vi "UT_FFTW.vi"(7 "UT FFTW States":T1=enum."Transform", 11 "Array":sgl[][](array[numeric])) -> (0 "Error":bool, 3 "Results":sgl[][](array[numeric]))   [LabVIEW 2014]
uses:
  UT FFTW States.ctl
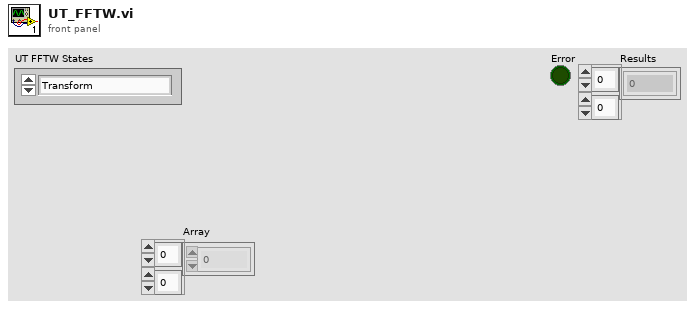
[diagram p1: front panel]
types:
  T1 = typedef "UT FFTW States.ctl" = enum16{"Init", "Transform", "Cleanup"}
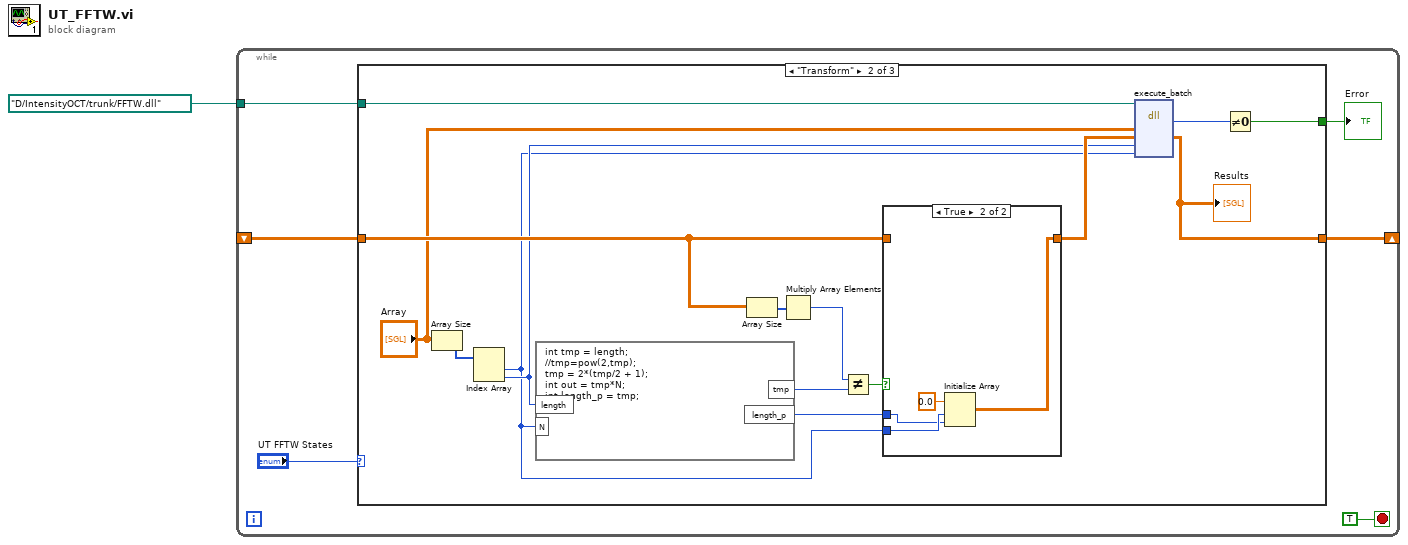
[diagram p0: block diagram]
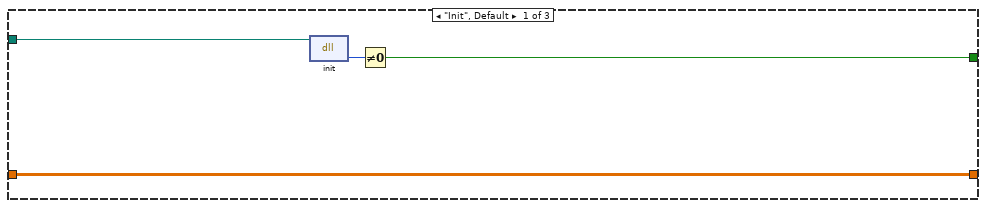
[diagram p2: hidden frame]
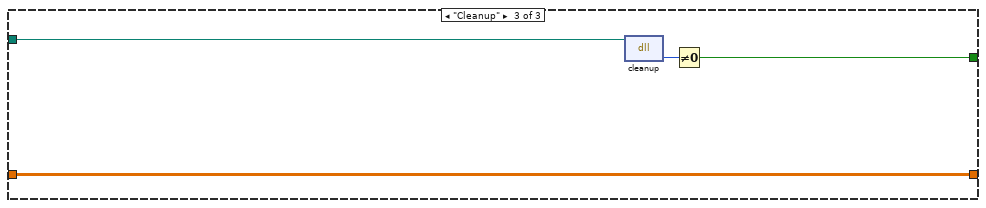
[diagram p4: hidden frame]
diagram:
  n1 = while {
    tunnel: path "D:/IntensityOCT/trunk/FFTW.dll" ("path in") -> [w5]
    shift-right: [w2] -> _
    shift-left: _ -> [w3]
    stop <- TRUE stop-if-true
    n2 = case shown="\"Transform\"" "UT FFTW States" {
      tunnel: w5 -> [w11 w19 w34]
      tunnel: [w9 w15 w32] -> w4
      tunnel: w3 -> [w8 w21 w35]
      tunnel: [w8 w14 w35] -> w2
      frame "Init", Default {
        n3 = dll-call lib="D:/IntensityOCT/trunk/FFT_CPP/x64/Release DLL/FFTW.dll" fn="init"(path in=w11) -> ("return type"=w10:i32)  [unwired: 2 in, 2 out]
        n4 = Not Equal To 0?(x=w10) -> (x != 0?=w9:bool)
      }
      frame "Transform" {
        n5 = Array Size(array="Array") -> (size(s)=w26:i32[])
        n6 = Index Array(array=w26) -> (element #1=w12:i32, element #2=w13:i32)  [unwired: 2 in]
        n7 = formula code="int tmp = length;\n//tmp=pow(2,tmp);\ntmp = 2*(tmp/2 + 1);\nint out = tmp*N;\nint length_p = tmp;"("length"=w13, "N"=w12) -> ("tmp"=w24:i32, "length_p"=w20:i32)
        n8 = Array Size(array=w21) -> (size(s)=w25:i32[])
        n9 = Multiply Array Elements(1:w25) -> (0:w23:i32)
        n10 = Not Equal?(x=w23, y=w24) -> (x != y?=w22:bool)
        n11 = case shown="True" w22 {
          tunnel: w21 -> [w27 _]
          tunnel: [w27 w31] -> w18
          tunnel: w20 -> [_ w28]
          tunnel: w12 -> [_ w29]
          frame False {
          }
          frame True {
            n12 = Initialize Array(sgl 0.0 ("element"), w29, w28) -> (w31:sgl[][])
          }
        }
        n13 = dll-call lib="D:/IntensityOCT/trunk/FFT_CPP/x64/Release DLL/FFTW.dll" fn="execute_batch"(path in=w19, "in"="Array", "out"=w18, "Length"=w13, "N"=w12) -> ("return type"=w16:i32, "out"=w14:sgl[][])  [unwired: 5 in, 2 out]
        "Results" <- w14
        n14 = Not Equal To 0?(x=w16) -> (x != 0?=w15:bool)
      }
      frame "Cleanup" {
        n15 = dll-call lib="D:/IntensityOCT/trunk/FFT_CPP/x64/Release DLL/FFTW.dll" fn="cleanup"(path in=w34) -> ("return type"=w33:i32)  [unwired: 2 in, 2 out]
        n16 = Not Equal To 0?(x=w33) -> (x != 0?=w32:bool)
      }
    }
    "Error" <- w4
  }
